vi "Get Speciality IO Raw Data.vi"() -> ()   [LabVIEW 2018]
uses:
  NiFpga.dll
panel:
  out "U8":u32
  out "i16":i16
  out "error code":i32
  in  "stop":bool
  out "FXP Value":dbl
  out "error out":errorcluster
  in  "Error In":errorcluster
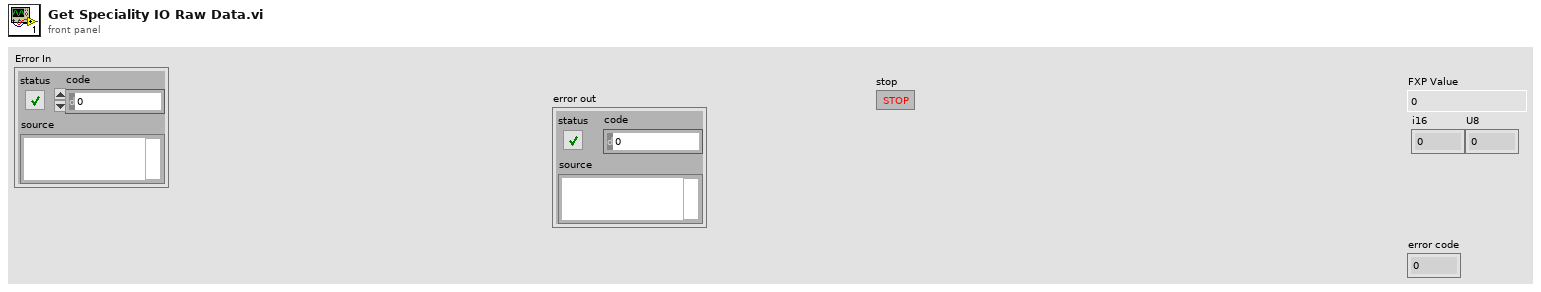
[diagram p1: front panel]
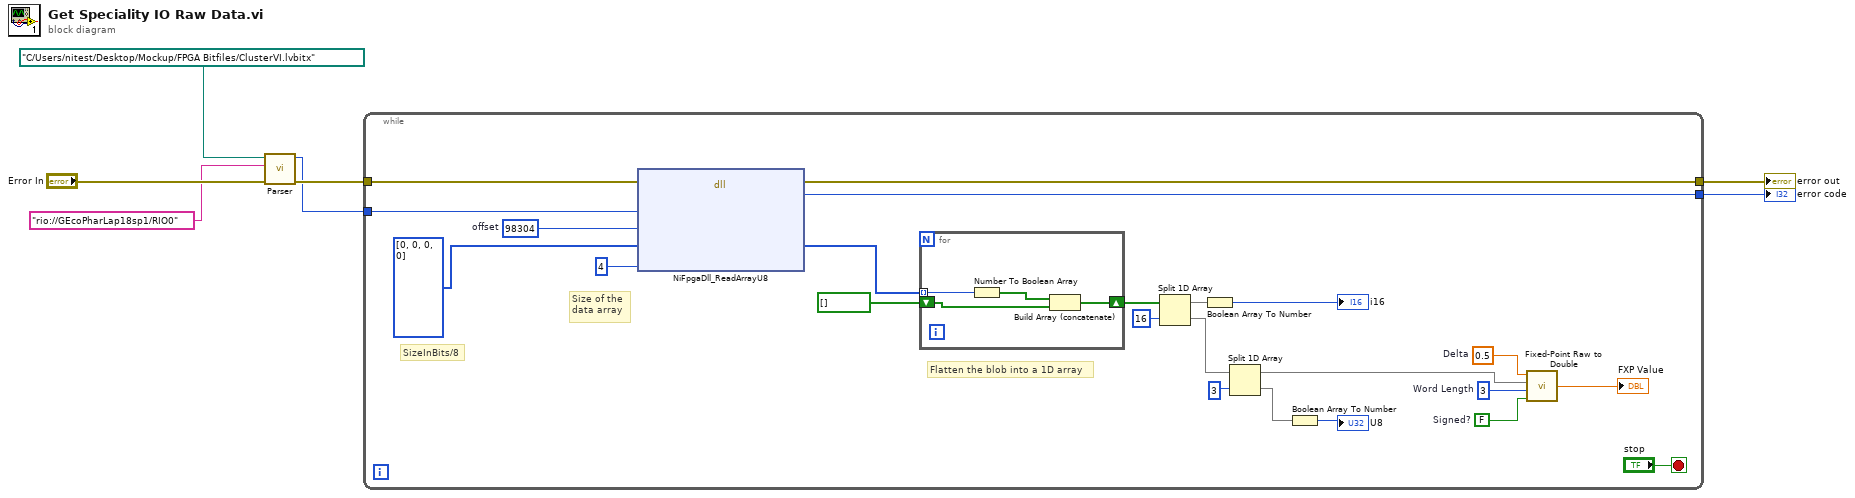
[diagram p0: block diagram]
diagram:
  n1 = call "Parser.vi"("error in (no error)"="Error In", "RIO device address"="rio://GEcoPharLap18sp1/RIO0" ("Device address"), "bitfile path"=path "C:/Users/nitest/Desktop/Mockup/FPGA Bitfiles/ClusterVI.lvbitx" ("Bitfile path")) -> ("error out"=w5:errorcluster, "session out"=w3:u64)  [unwired: 6 in, 1 out]
  n2 = while {
    tunnel: w5 -> [w30]
    tunnel: w3 -> [w29]
    tunnel: [w9] -> w2
    tunnel: [w8] -> w1
    stop <- "stop" stop-if-true
    w21 = FALSE  # Signed?
    w22 = u8 3  # Word Length
    w23 = 0.5  # Delta
    w28 = u32 98304  # offset
    # "Flatten the blob into a 1D array"
    # "Size of the \ndata array"
    # "SizeInBits/8"
    n3 = dll-call lib="NiFpga.*" fn="NiFpgaDll_ReadArrayU8"(error in=w30, "session"=w29, "offset"=w28, "data"=u8[] [0, 0, 0, 0], "count"=u8 4) -> (error out=w9:errorcluster, "status"=w8:i32, "data"=w25:u8[])  [unwired: 5 in, 1 out]
    n4 = for {
      shift-right: [w32] -> w19
      shift-left: bool[] [] ("element") -> [w33]
      tunnel: w25 -> [w31] mode=indexing
      n5 = Number To Boolean Array(number=w31) -> (Boolean array=w34:bool[])
      n6 = Build Array (concatenate)(w34, w33) -> (w32:bool[])
    }
    n7 = Split 1D Array(array=w19, index=16) -> (first subarray=w14:bool[], second subarray=w16:bool[])
    n8 = Boolean Array To Number(Boolean array=w14) -> (number=→"i16":u32)
    n9 = Split 1D Array(array=w16, index=3) -> (first subarray=w11:bool[], second subarray=w10:bool[])
    n10 = Boolean Array To Number(Boolean array=w10) -> (number=→"U8":u32)
    n11 = call "Fixed-Point Raw to Double.vi"("Signed?"=w21, "Word Length"=w22, "Data"=w11, "Delta"=w23) -> ("value"=→"FXP Value":dbl)
  }
  "error out" <- w2
  "error code" <- w1
